vi "OnshapeConnection.vi"() -> ()   [LabVIEW 2024]
uses:
  <vilib>/Analysis/Matrix/Datatypes/RealMatrix.ctl
  <vilib>/Analysis/baseanly.llb/Real A x B.vi
  <vilib>/httpClient/LabVIEWHTTPClient.lvlib
  <vilib>/Utility/SMTP/NI_SMTPEmail.lvlib
  <vilib>/Analysis/Matrix/NI_Matrix.lvlib
  <vilib>/Analysis/NI_AALBase.lvlib
panel:
  in  "Array":T1(array[cluster])=[{"Translation"={"X"=0.0, "Y"=0.0, "Z"=6.0}, "Axis"=enum."z", "Angle (degrees)"=0.0, "variable?"=FALSE}, {"Translation"={"X"=0.0, "Y"=0.0, "Z"=0.0}, "Axis"=enum."y", "Angle (degrees)"=90.0, "variable?"=FALSE}, {"Translation"={"X"=0.0, "Y"=0.0, "Z"=5.0}, "Axis"=enum."z", "Angle (degrees)"=-90.0, "variable?"=FALSE}, {"Translation"={"X"=0.0, "Y"=0.0, "Z"=0.0}, "Axis"=enum."z", "Angle (degrees)"=0.0, "variable?"=FALSE}, {"Translation"={"X"=10.0, "Y"=0.0, "Z"=0.0}, "Axis"=enum."z", "Angle (degrees)"=0.0, "variable?"=FALSE}, {"Translation"={"X"=0.0, "Y"=0.0, "Z"=-3.5}, "Axis"=enum."z", "Angle (degrees)"=0.0, "variable?"=FALSE}, {"Translation"={"X"=8.0, "Y"=0.0, "Z"=0.0}, "Axis"=enum."z", "Angle (degrees)"=0.0, "variable?"=FALSE}, {"Translation"={"X"=0.0, "Y"=0.0, "Z"=4.5}, "Axis"=enum."x", "Angle (degrees)"=-90.0, "variable?"=FALSE}, {"Translation"={"X"=0.0, "Y"=0.0, "Z"=3.0}, "Axis"=enum."z", "Angle (degrees)"=0.0, "variable?"=FALSE}, {"Translation"={"X"=0.0, "Y"=0.0, "Z"=0.0}, "Axis"=enum."x", "Angle (degrees)"=90.0, "variable?"=FALSE}, {"Translation"={"X"=0.0, "Y"=0.0, "Z"=4.0}, "Axis"=enum."z", "Angle (degrees)"=0.0, "variable?"=FALSE}] {"Angle (degrees)" scale=-90.0..90.0}
  out "3D Picture":refnum<vi>(3d-picture)
  out "Angles (deg)":dbl[](array[numeric])
  out "Angles (rad)":dbl[](array[numeric])
  out "URL  sent":string="https://cad.onshape.com/api/v10/assemblies/d/040c8fd429b5d751ae5dfd45/w/5b62e7d426c0ebc6d7945848/e/20ffb64d425fd3df0e20b281/matevalues"
  out "mateValues":T2(array[cluster])
  out "body":string
  out "headers":string
  # "base"
  # "shoulder"
  # "elbow"
  # "wrist1"
  # "wrist2"
  # "wrist3"
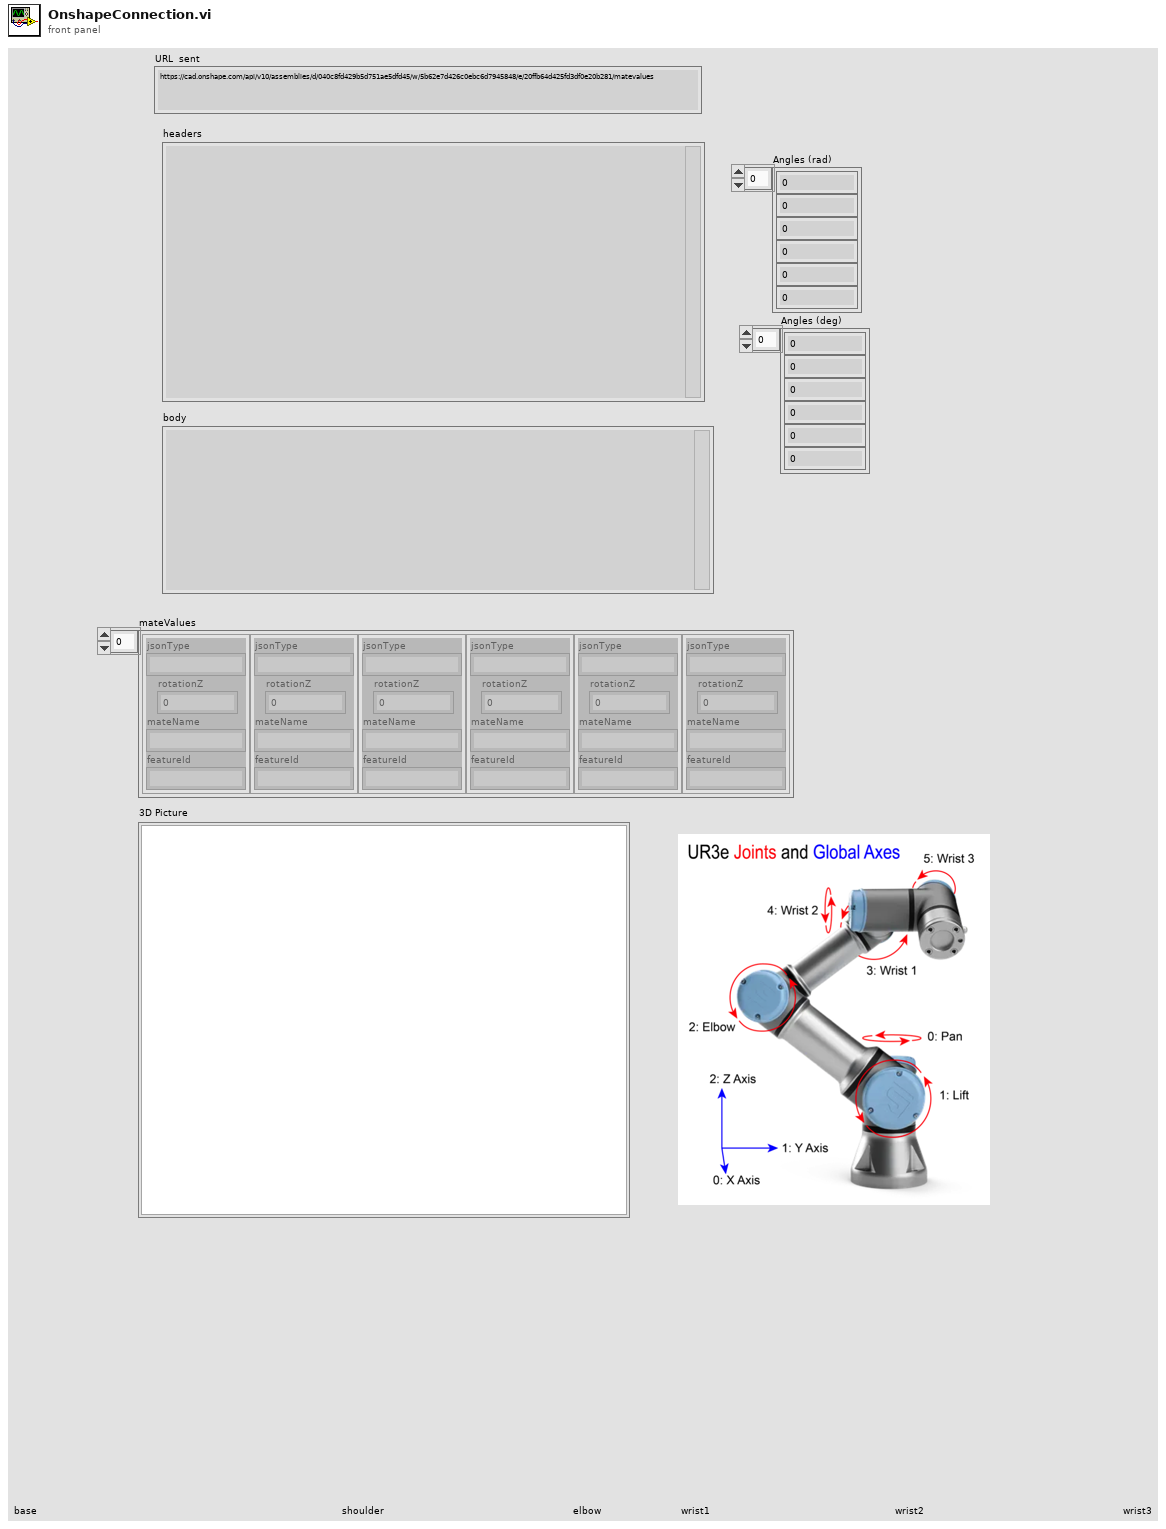
[diagram p1: front panel]
types:
  T1 = cluster{"Translation":cluster{"X":dbl, "Y":dbl, "Z":dbl}, "Axis":enum16{"x", "y", "z"}, "Angle (degrees)":dbl, "variable?":bool}[]
  T2 = cluster{"jsonType":string, "rotationZ":dbl, "mateName":string, "featureId":string}[]
  T3 = cluster{"mateValues":cluster{"jsonType":string, "rotationZ":dbl, "mateName":string, "featureId":string}[]}
  T4 = cluster{"Line width":sgl, "Line Color":u32, "Axes?":bool}
  T5 = typedef "NI_Matrix.lvlib/RealMatrix.ctl" = dbl[][]
  T6 = typedef "LabVIEWHTTPClient.lvlib/ClientHandle.ctl" = refnum<k1>
  T7 = cluster{"Translation":cluster{"X":dbl, "Y":dbl, "Z":dbl}, "Axis":enum16{"x", "y", "z"}, "Angle (degrees)":dbl, "variable?":bool}
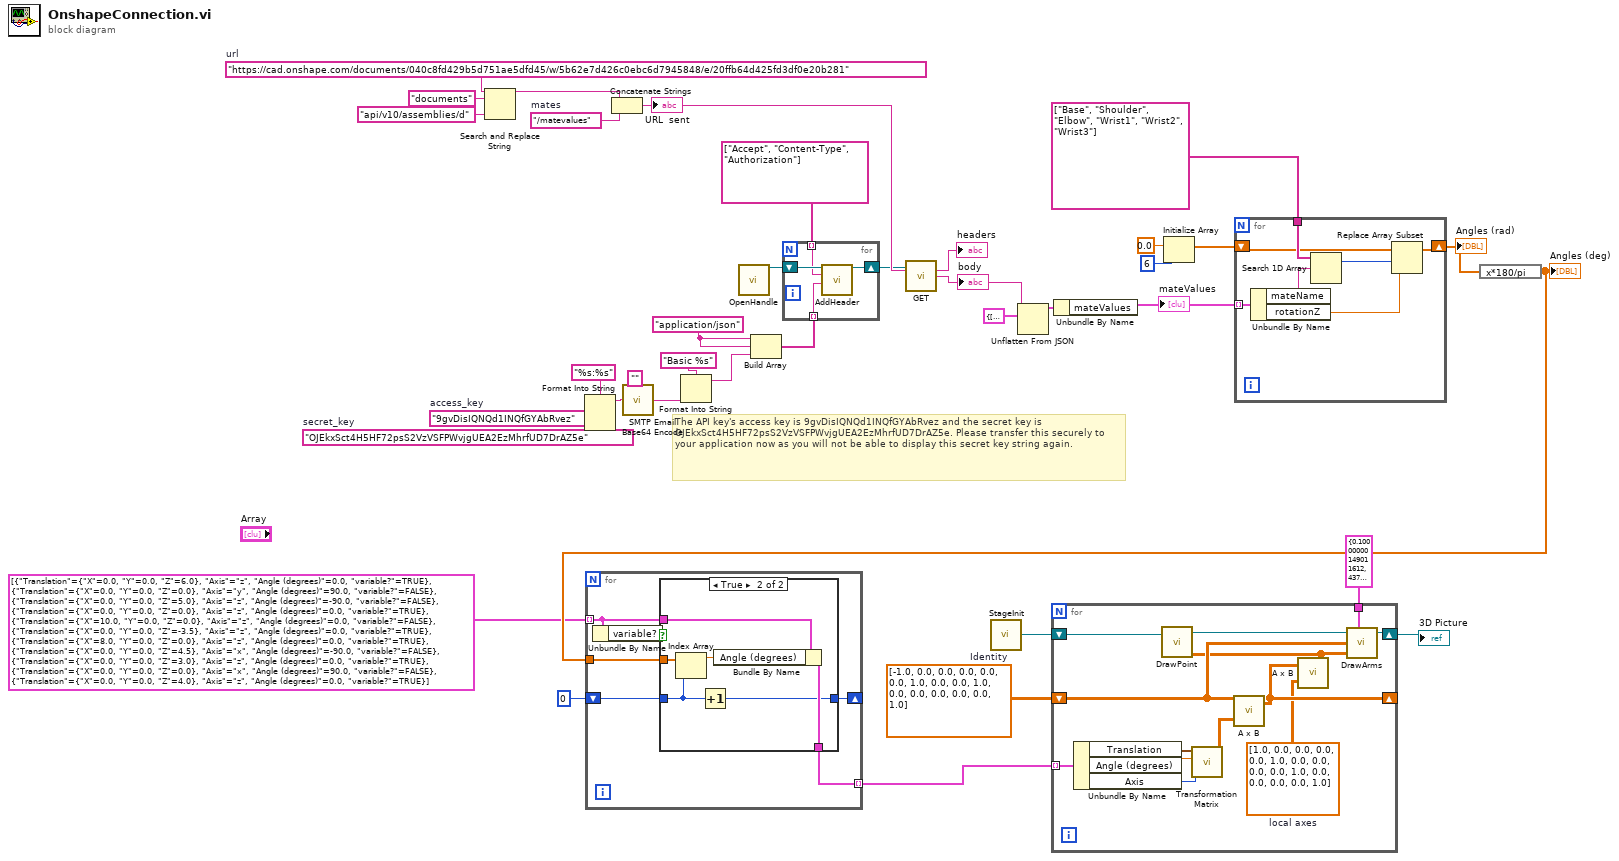
[diagram p0: block diagram]
diagram:
  w10 = "application/json" ("value")
  w20 = T5 [[-1.0, 0.0, 0.0, 0.0], [0.0, 0.0, 1.0, 0.0], [0.0, 1.0, 0.0, 0.0], [0.0, 0.0, 0.0, 1.0]]  # Identity
  w28 = "/matevalues"  # mates
  w35 = "OJEkxSct4H5HF72psS2VzVSFPWvjgUEA2EzMhrfUD7DrAZ5e"  # secret_key
  w36 = "9gvDisIQNQd1INQfGYAbRvez"  # access_key
  w32 = "https://cad.onshape.com/documents/040c8fd429b5d751ae5dfd45/w/5b62e7d426c0ebc6d7945848/e/20ffb64d425fd3df0e20b281"  # url
  # "The API key's access key is 9gvDisIQNQd1INQfGYAbRvez and the secret key is OJEkxSct4H5HF72psS2VzVSFPWvjgUEA2EzMhrfUD7DrAZ5e. Please transfer this securely to your application now as you will not be able to display this secret key string again."
  n1 = Search and Replace String(input string=w32, search string="documents", replace string="api/v10/assemblies/d" ("replace string (\"\")")) -> (result string=w29:string)  [unwired: 5 in, 3 out]
  n2 = Format Into String(format string="%s:%s", w36, w35) -> (resulting string=w34:string)  [unwired: 2 in, 1 out]
  n3 = Concatenate Strings(w29, w28) -> (w27:string)
  "URL  sent" <- w27
  n4 = call <vilib>:"SMTP Email Base64 Encode.vi"("Normal String"=w34, "Line separator (\\n)"="" ("Line separator (\\n)")) -> ("Base64 String"=w7:string)
  n5 = Format Into String(format string="Basic %s", w7) -> (resulting string=w6:string)  [unwired: 2 in, 1 out]
  n6 = call <vilib>:"OpenHandle.vi"() -> ("client handle out"=w11:T6)  [unwired: 14 in, 1 out]
  n7 = Build Array(w10, w10, w6) -> (w9:string[])
  n8 = for {
    shift-right: [w41] -> w12
    shift-left: w11 -> [w40]
    tunnel: string[] ["Accept", "Content-Type", "Authorization"] -> [w39] mode=indexing
    tunnel: w9 -> [w38] mode=indexing
    n9 = call <vilib>:"AddHeader.vi"("client handle"=w40, "header"=w39, "value"=w38) -> ("client handle out"=w41:T6)  [unwired: 11 in, 1 out]
  }
  n10 = call <vilib>:"GET.vi"("client handle"=w12, "url"=w27) -> ("headers"=→"headers":string, "body"=w5:string)  [unwired: 10 in, 2 out]
  "body" <- w5
  n11 = call <userlib>:"StageInit.vi"() -> ("Stage out"=w18:refnum<vi>)  [unwired: 4 in, 1 out]
  n12 = Unflatten From JSON(JSON string=w5, type and defaults=T3 {"mateValues"=[{"jsonType"="", "rotationZ"=0.0, "mateName"="", "featureId"=""}]}) -> (value=w3:T3)  [unwired: 5 in, 1 out]
  n13 = Unbundle By Name(w3) -> ("mateValues"=w26:T2)
  "mateValues" <- w26
  n14 = Initialize Array(0.0 ("element"), 6 ("dimension size")) -> (w23:dbl[])
  n15 = for {
    tunnel: w26 -> [w48] mode=indexing
    shift-right: [w45] -> w21
    shift-left: w23 -> [w44]
    tunnel: string[] ["Base", "Shoulder", "Elbow", "Wrist1", "Wrist2", "Wrist3"] -> [w46]
    n16 = Unbundle By Name(w48) -> ("mateName"=w47:string, "rotationZ"=w42:dbl)
    n17 = Search 1D Array(1D array=w46, element=w47) -> (index of element=w43:i32)  [unwired: 1 in]
    n18 = Replace Array Subset(array=w44, new element=w42, index=w43) -> (w45:dbl[])
  }
  "Angles (rad)" <- w21
  n19 = expression code="x*180/pi"(w21) -> (w16:dbl[])
  "Angles (deg)" <- w16
  n20 = for {
    tunnel: w16 -> [w53]
    tunnel: T1 [{"Translation"={"X"=0.0, "Y"=0.0, "Z"=6.0}, "Axis"=enum."z", "Angle (degrees)"=0.0, "variable?"=TRUE}, {"Translation"={"X"=0.0, "Y"=0.0, "Z"=0.0}, "Axis"=enum."y", "Angle (degrees)"=90.0, "variable?"=FALSE}, {"Translation"={"X"=0.0, "Y"=0.0, "Z"=5.0}, "Axis"=enum."z", "Angle (degrees)"=-90.0, "variable?"=FALSE}, {"Translation"={"X"=0.0, "Y"=0.0, "Z"=0.0}, "Axis"=enum."z", "Angle (degrees)"=0.0, "variable?"=TRUE}, {"Translation"={"X"=10.0, "Y"=0.0, "Z"=0.0}, "Axis"=enum."z", "Angle (degrees)"=0.0, "variable?"=FALSE}, {"Translation"={"X"=0.0, "Y"=0.0, "Z"=-3.5}, "Axis"=enum."z", "Angle (degrees)"=0.0, "variable?"=TRUE}, {"Translation"={"X"=8.0, "Y"=0.0, "Z"=0.0}, "Axis"=enum."z", "Angle (degrees)"=0.0, "variable?"=TRUE}, {"Translation"={"X"=0.0, "Y"=0.0, "Z"=4.5}, "Axis"=enum."x", "Angle (degrees)"=-90.0, "variable?"=FALSE}, {"Translation"={"X"=0.0, "Y"=0.0, "Z"=3.0}, "Axis"=enum."z", "Angle (degrees)"=0.0, "variable?"=TRUE}, {"Translation"={"X"=0.0, "Y"=0.0, "Z"=0.0}, "Axis"=enum."x", "Angle (degrees)"=90.0, "variable?"=FALSE}, {"Translation"={"X"=0.0, "Y"=0.0, "Z"=4.0}, "Axis"=enum."z", "Angle (degrees)"=0.0, "variable?"=TRUE}] ("Array") -> [w52] mode=indexing
    tunnel: [w54] -> w2 mode=indexing
    shift-right: [w49] -> _
    shift-left: 0 -> [w50]
    n21 = Unbundle By Name(w52) -> ("variable?"=w51:bool)
    n22 = case shown="True" w51 {
      tunnel: [w55 w62] -> w54
      tunnel: w53 -> [_ w61]
      tunnel: w52 -> [w55 w59]
      tunnel: w50 -> [w56 w58]
      tunnel: [w56 w57] -> w49
      frame False {
      }
      frame True {
        n23 = Index Array(array=w61, index=w58) -> (element=w60:dbl)
        n24 = Increment(x=w58) -> (x+1=w57:i32)
        n25 = Bundle By Name(cluster=w59, "Angle (degrees)"=w60) -> (w62:T7)
      }
    }
  }
  n26 = for {
    tunnel: w2 -> [w75] mode=indexing
    shift-right: [w68] -> _
    shift-left: w20 -> [w65]
    tunnel: T4 {"Line width"=0.1, "Line Color"=4376575, "Axes?"=TRUE} ("Params") -> [w70]
    shift-right: [w69] -> w17
    shift-left: w18 -> [w66]
    w67 = T5 [[1.0, 0.0, 0.0, 0.0], [0.0, 1.0, 0.0, 0.0], [0.0, 0.0, 1.0, 0.0], [0.0, 0.0, 0.0, 1.0]]  # local axes
    n27 = Unbundle By Name(w75) -> ("Translation"=w74:cluster{"X":dbl, "Y":dbl, "Z":dbl}, "Angle (degrees)"=w73:dbl, "Axis"=w72:enum16{"x", "y", "z"})
    n28 = call <userlib>:"Transformation Matrix.vi"("Axis"=w72, "Angle (degrees)"=w73, "Translation"=w74) -> ("Transformation Matrix"=w71:T5)  [unwired: 8 in]
    n29 = call-poly <vilib>:"A x B.vi"("B"=w71, "A"=w65) -> ("A x B"=w68:T5)  [unwired: 1 out]
    n30 = call-poly <vilib>:"A x B.vi"("B"=w67, "A"=w68) -> ("A x B"=w63:T5)  [unwired: 1 out]
    n31 = call <userlib>:"DrawPoint.vi"("Start"=w63, "Stage in"=w66) -> ("Stage out"=w64:refnum<vi>)  [unwired: 1 in]
    n32 = call <userlib>:"DrawArms.vi"("Stage in"=w64, "Params"=w70, "Start"=w65, "End"=w63) -> ("Stage out"=w69:refnum<vi>)  [unwired: 2 in, 1 out]
  }
  "3D Picture" <- w17
